vi "Rolling Average.vi"(11 "Neue Messwerte":sgl[](array[numeric])) -> (1 "Rolling Average":sgl[](array[numeric]), 3 "Aktuelle Messwerte":sgl[](array[numeric]))   [LabVIEW 2020, in "Messdaten.lvlib"]
uses:
  Messdaten.lvlib
  Gewichtung (Stichprobe).ctl
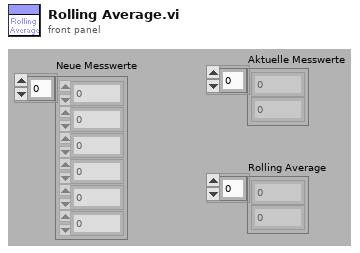
[diagram p1: front panel]
types:
  T1 = typedef "Messdaten.lvlib/Gewichtung (Stichprobe).ctl" = enum16{"Sample", "Population"}
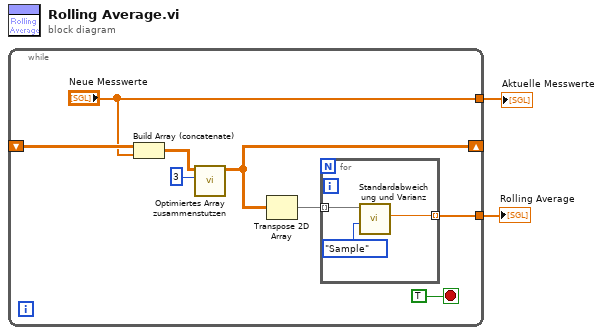
[diagram p0: block diagram]
diagram:
  n1 = while {
    shift-right: [w4] -> _
    shift-left: _ -> [w9]
    tunnel: [w6] -> w2
    tunnel: ["Neue Messwerte"] -> w1
    stop <- TRUE stop-if-true
    n2 = Build Array (concatenate)(w9, "Neue Messwerte") -> (w7:sgl[][])
    n3 = call "Optimiertes Array zusammenstutzen.vi"("Anzahl Elemente"=3, "Messdaten"=w7) -> ("Messdaten"=w4:sgl[][])  [unwired: 8 in, 1 out]
    n4 = Transpose 2D Array(2D array=w4) -> (transposed array=w3:sgl[][])
    n5 = for {
      tunnel: w3 -> [w13] mode=indexing
      tunnel: [w11] -> w6 mode=indexing
      n6 = call "Standardabweichung und Varianz.vi"("Gewichtung (Stichprobe)"=Gewichtung_(Stichprobe)."Sample", "X"=w13) -> ("Mittelwert"=w11:sgl)  [unwired: 7 in, 2 out]
    }
  }
  "Aktuelle Messwerte" <- w1
  "Rolling Average" <- w2
